vi "Logging Settings Window.vi"(8 "Error In":errorcluster) -> (0 "Error Out":errorcluster)   [LabVIEW 2019]
uses:
  Controls/Logging Settings.ctl
panel:
  in  "Logging Settings":T1={"Logging Interval [s]"=1.0, "Use Lowpass Filter"=TRUE, "Tf [s]"=5.0, "Logging Data to File"=TRUE, "Log Folder"=path "c:/Temp/Data.lvm", "Logging Data to Cloud Service"=FALSE, "Data Cloud Service Url"="http://127.0.0.1:8001/DataWS", "Use Random Data"=TRUE}
  in  "Cancel Button":bool
  in  "OK Button":bool
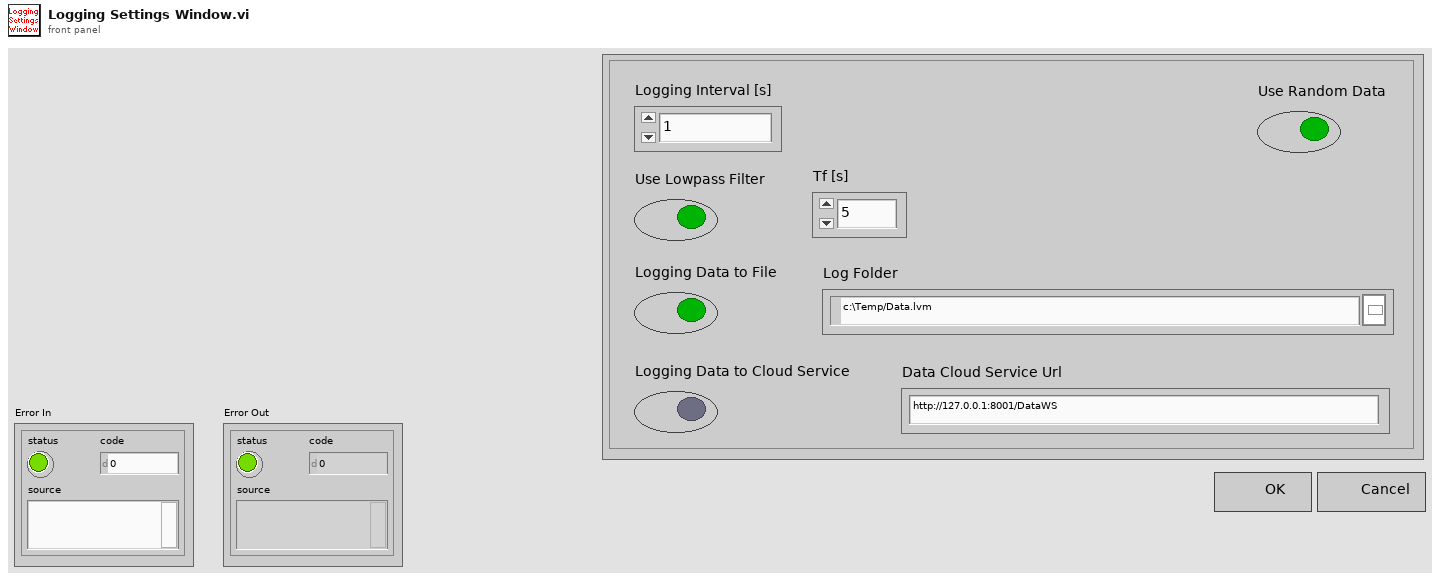
[diagram p1: front panel]
types:
  T1 = typedef "Logging Settings.ctl" = cluster{"Logging Interval [s]":dbl, "Use Lowpass Filter":bool, "Tf [s]":dbl, "Logging Data to File":bool, "Log Folder":path, "Logging Data to Cloud Service":bool, "Data Cloud Service Url":string, "Use Random Data":bool}
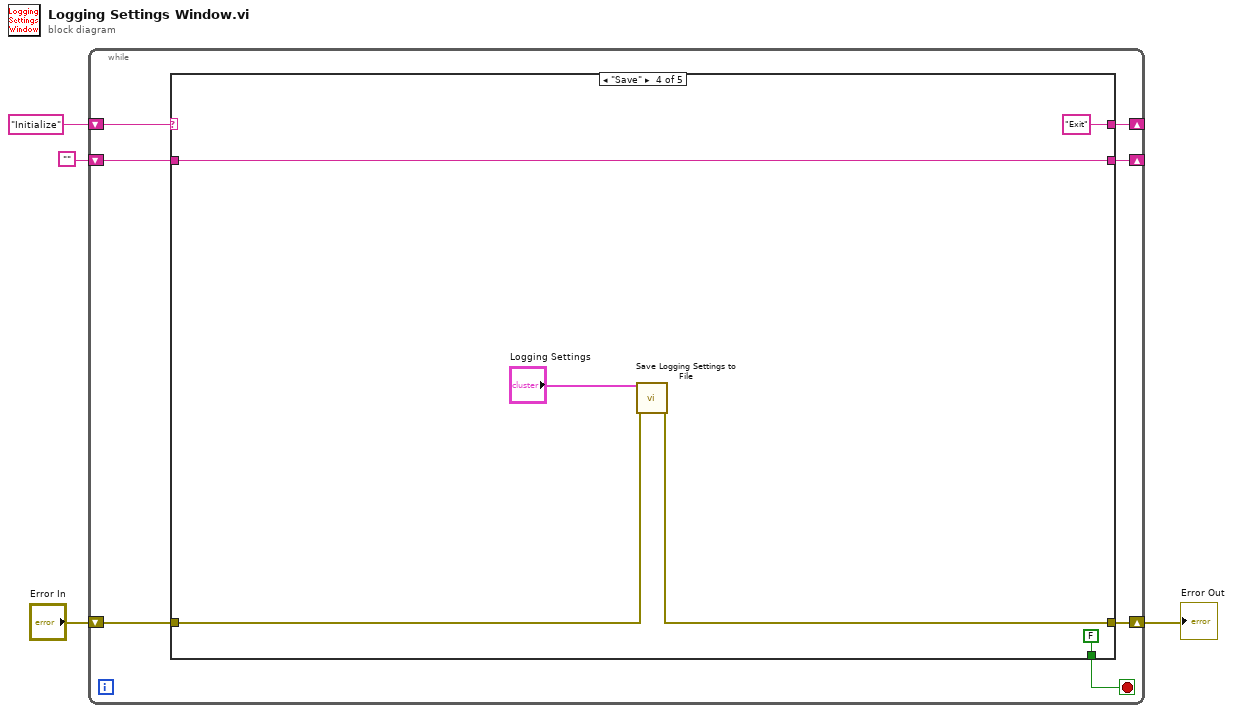
[diagram p0: block diagram]
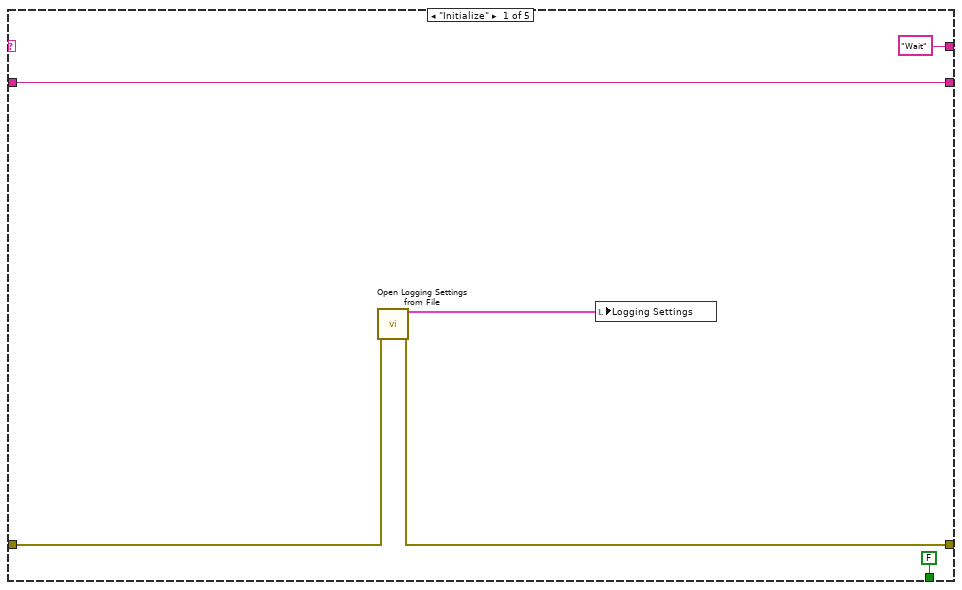
[diagram p2: hidden frame]
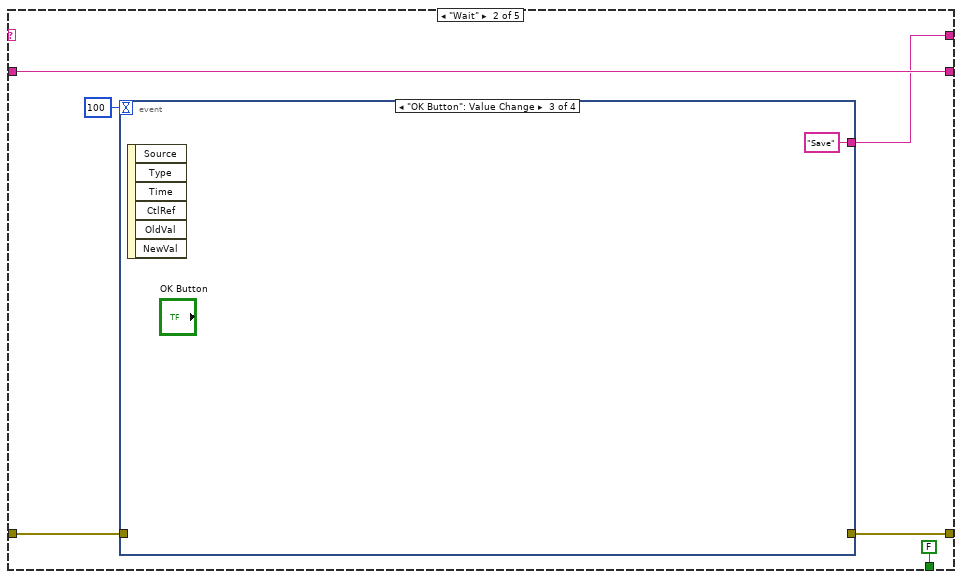
[diagram p3: hidden frame]
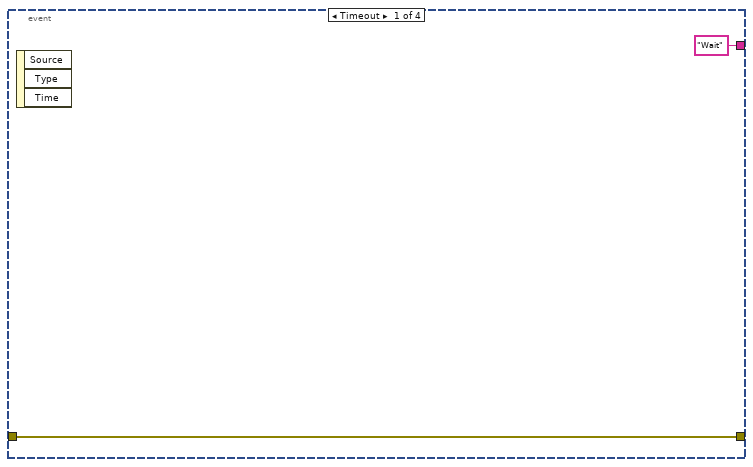
[diagram p4: hidden frame]
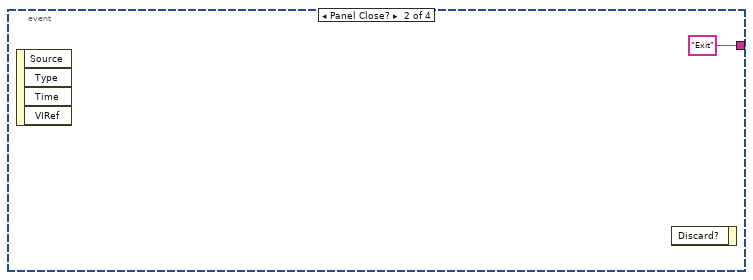
[diagram p5: hidden frame]
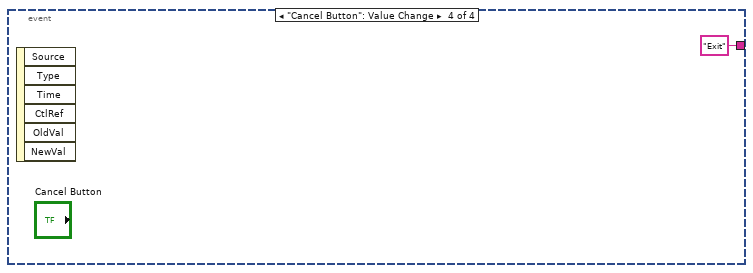
[diagram p6: hidden frame]
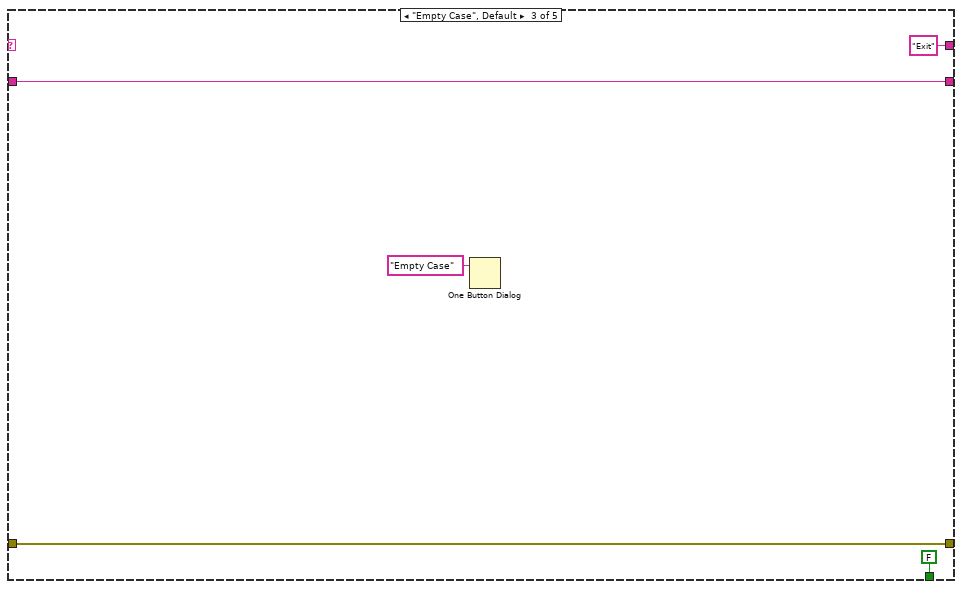
[diagram p7: hidden frame]
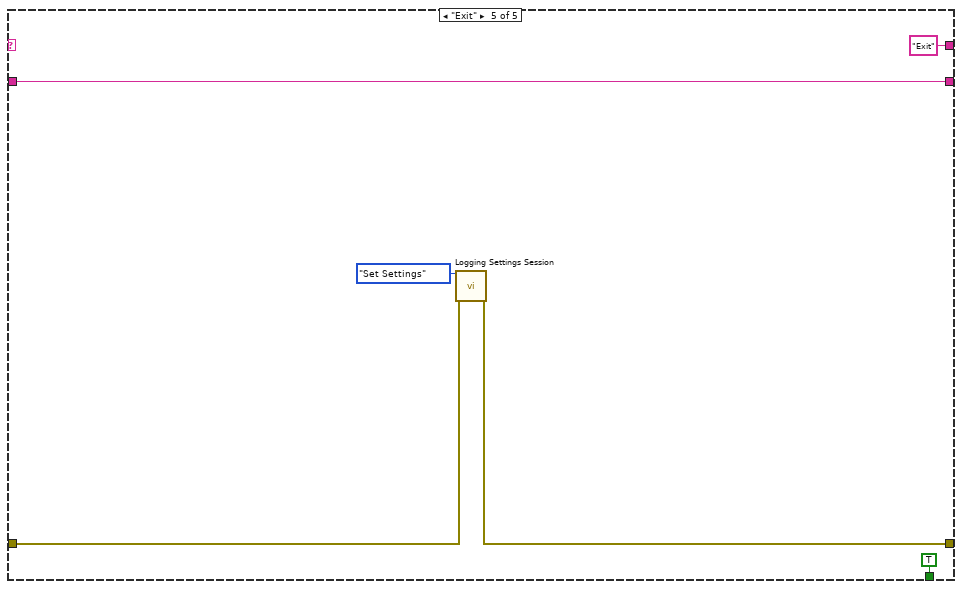
[diagram p8: hidden frame]
diagram:
  n1 = while {
    shift-right: [w7] -> _
    shift-left: "Initialize" ("key") -> [w11]
    shift-right: [w8] -> _
    shift-left: "" -> [w10]
    shift-right: [w5] -> w2
    shift-left: "Error In" -> [w9]
    stop <- w6 stop-if-true
    n2 = case shown="\"Save\"" w11 {
      tunnel: w10 -> [w15 w22 w30 w37 w45]
      tunnel: w9 -> [w13 w19 w31 w35 w41]
      tunnel: [w15 w22 w30 w37 w45] -> w8
      tunnel: ["Wait" ("key") w21 "Exit" ("key") "Exit" ("key") "Exit" ("key")] -> w7
      tunnel: [FALSE FALSE FALSE FALSE TRUE] -> w6
      tunnel: [w12 w18 w31 w34 w40] -> w5
      frame "Initialize" {
        n3 = call "Open Logging Settings from File.vi"("Error In"=w13) -> ("Logging Settings"=w14:T1, "Error Out"=w12:errorcluster)  [unwired: 13 in]
        n4 = local write "Logging Settings"(w14) -> ()
      }
      frame "Wait" {
        n5 = event shown="[2] \"OK Button\": Value Change" {
          selector: _ -> [_ _ _ _]
          dyn-events: _ -> [_ _ _ _]
          timeout: 100 -> [_ _ _ _]
          tunnel: ["Wait" ("key") "Exit" ("key") "Save" ("key") "Exit" ("key")] -> w21
          tunnel: w19 -> [w24 _ _ _]
          tunnel: [w24 _ _ _] -> w18
          event Timeout {
            n6 = event-data() -> ()  [unwired: 1 in, 3 out]
          }
          event Panel Close? {
            n7 = event-data() -> ()  [unwired: 1 in, 4 out]
            n8 = event-data() -> ()  [unwired: 2 in, 1 out]
          }
          event "OK Button": Value Change {
            n9 = event-data() -> ()  [unwired: 1 in, 6 out]
          }
          event "Cancel Button": Value Change {
            n10 = event-data() -> ()  [unwired: 1 in, 6 out]
          }
        }
      }
      frame "Empty Case", Default {
        n11 = One Button Dialog(message="Empty Case") -> ()  [unwired: 1 in, 1 out]
      }
      frame "Save" {
        n12 = call "Save Logging Settings to File.vi"("Logging Settings"="Logging Settings", "Error In"=w35) -> ("Error Out"=w34:errorcluster)  [unwired: 13 in]
      }
      frame "Exit" {
        n13 = call "Logging Settings Session.vi"("Type"=enum16{"Set Settings", "Get Settings"}."Set Settings", "Error In"=w41) -> ("Error Out"=w40:errorcluster)  [unwired: 12 in, 1 out]
      }
    }
  }
  "Error Out" <- w2
